vi "Write UI VI.vi"(8 "error in (no error)":errorcluster, 10 "UI VI":refnum<vi>, 11 "UI CMD in":refnum<class "UI CMD.lvclass">) -> (0 "error out":errorcluster, 3 "UI CMD out":refnum<class "UI CMD.lvclass">)   [LabVIEW 2014, in "UI CMD.lvclass"]
uses:
  UI CMD.lvclass
  UI CMD.lvclass/UI CMD.ctl
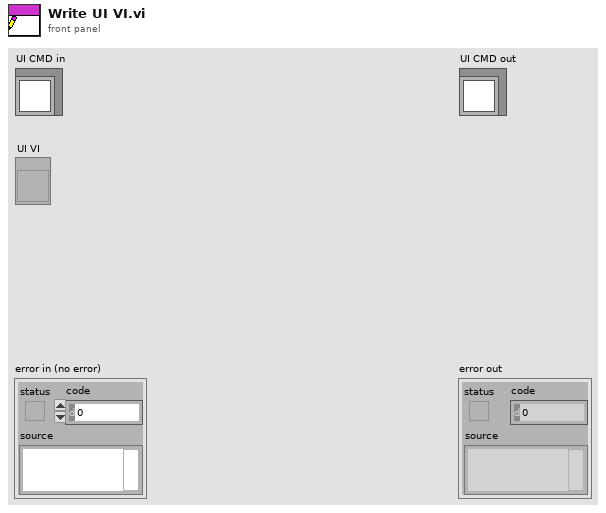
[diagram p1: front panel]
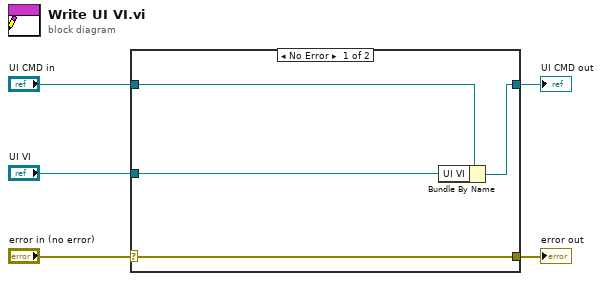
[diagram p0: block diagram]
diagram:
  n1 = case shown="No Error" "error in (no error)" {
    selector: "error in (no error)" -> [w9 w10]
    tunnel: [w9 w10] -> w4
    tunnel: [w7 w11] -> w2
    tunnel: "UI CMD in" -> [w8 w11]
    tunnel: "UI VI" -> [w6 _]
    frame No Error {
      n2 = Bundle By Name(cluster=w8, "UI VI"=w6) -> (w7:refnum<class "UI CMD.lvclass">)
    }
    frame Error {
    }
  }
  "error out" <- w4
  "UI CMD out" <- w2
